vi "Interpolation.vi"(2 "dt":dbl, 3 "Shifted Y":dbl[](array[numeric]), 4 "Original X":dbl[](array[numeric])) -> (0 "k":i32, 1 "Recovered Y":dbl[](array[numeric]))   [LabVIEW 2015]
uses:
  <vilib>/Analysis/NI_AALPro.lvlib
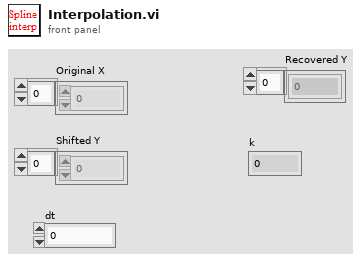
[diagram p1: front panel]
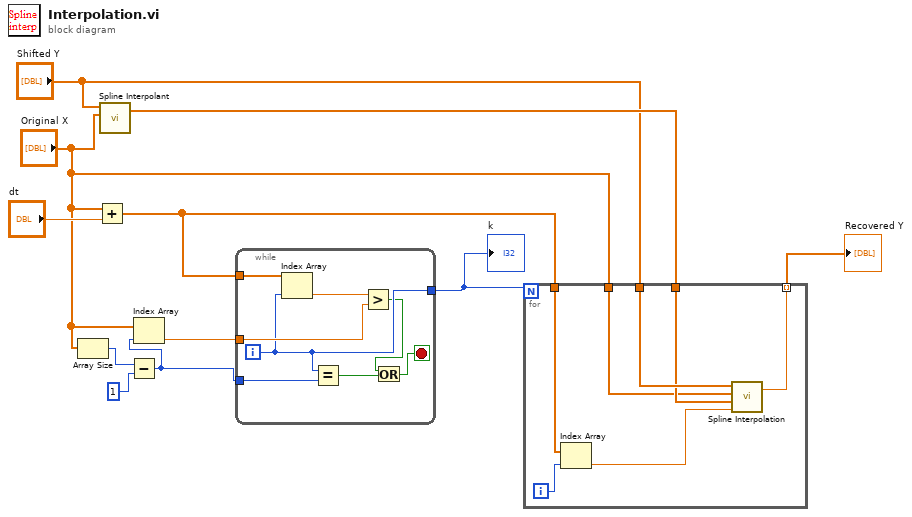
[diagram p0: block diagram]
diagram:
  n1 = Array Size(array="Original X") -> (size(s)=w4:i32)
  n2 = Add(x="Original X", y="dt") -> (x+y=w2:dbl[])
  n3 = call <vilib>:"Spline Interpolant.vi"("X"="Original X", "Y"="Shifted Y") -> ("Interpolant"=w9:dbl[])  [unwired: 2 in, 1 out]
  n4 = Subtract(x=w4, y=1) -> (x-y=w6:i32)
  n5 = Index Array(array="Original X", index=w6) -> (element=w5:dbl)
  n6 = while {
    tunnel: w2 -> [w19]
    tunnel: w5 -> [w17]
    tunnel: [w16] -> w3
    tunnel: w6 -> [w15]
    i -> [w16]
    stop <- w12 stop-if-true
    n7 = Index Array(array=w19, index=w16) -> (element=w18:dbl)
    n8 = Equal?(x=w16, y=w15) -> (x = y?=w14:bool)
    n9 = Greater?(x=w18, y=w17) -> (0:w13:bool)
    n10 = Or(x=w13, y=w14) -> (x .or. y?=w12:bool)
  }
  "k" <- w3
  n11 = for {
    N: w3 -> [_]
    tunnel: w2 -> [w26]
    tunnel: w9 -> [w21]
    tunnel: "Shifted Y" -> [w22]
    tunnel: [w24] -> w10 mode=indexing
    tunnel: "Original X" -> [w20]
    i -> [w23]
    n12 = Index Array(array=w26, index=w23) -> (element=w25:dbl)
    n13 = call <vilib>:"Spline Interpolation.vi"("x value"=w25, "Interpolant"=w21, "X"=w20, "Y"=w22) -> ("interpolation value"=w24:dbl)  [unwired: 1 out]
  }
  "Recovered Y" <- w10
